vi "MB Ethernet Example Master.vi"() -> ()   [LabVIEW 2019, in "NI_modbus_upd.lvlib"]
uses:
  NI_modbus_upd.lvlib
  Ctl/MB Modbus Command.ctl
  TCP/TCP.lvclass
panel:
  out "error out":errorcluster
  in  "Remote Port":u16=502
  in  "Remote IP Address":string="127.0.0.1"
  in  "Stop":bool
  out "Slave Input Registers":u16[](array[numeric]) caption="Slave Input Registers (Read Only)"
  out "Slave Discrete Inputs":bool[](array[boolean])
  in  "Coils to Write":bool[](array[boolean])=[FALSE, FALSE, FALSE, FALSE]
  in  "Registers to Write":u16[](array[numeric])=[0, 0, 0, 0]
  # "MB Ethernet Example Master.vi\n\nInstructions\n1. Run MB Ethernet Example Slave.vi\n2. Run this VI.\n3. Modify the discrete inputs or input registers on the slave -> they're updated on the master.\n4. Modify the coils and registers on the master -> they're updated on the slave."
  # "Data to write to the slave"
  # "Slave Read-only Registers"
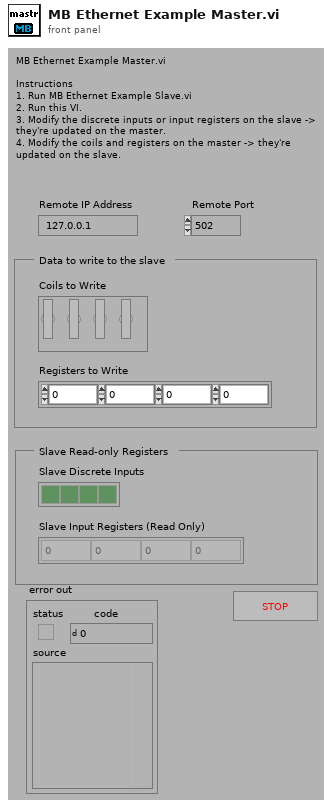
[diagram p1: front panel]
types:
  T1 = typedef "NI_modbus_upd.lvlib/MB Modbus Command.ctl" = cluster{"Function Code":u8, "Starting Address":u16, "Quantity":u16, "Data":u16[], "Discrete":bool[]}
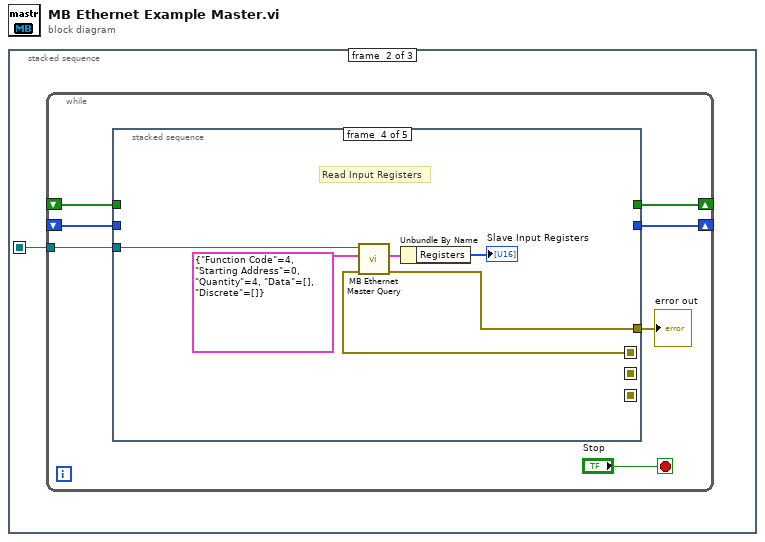
[diagram p0: block diagram]
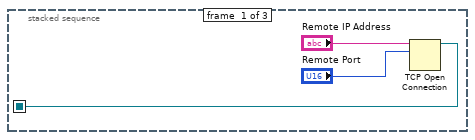
[diagram p2: hidden frame]
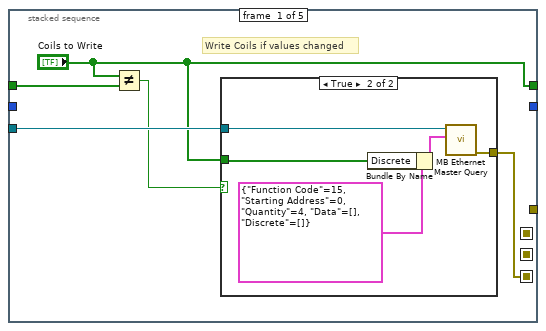
[diagram p3: hidden frame]
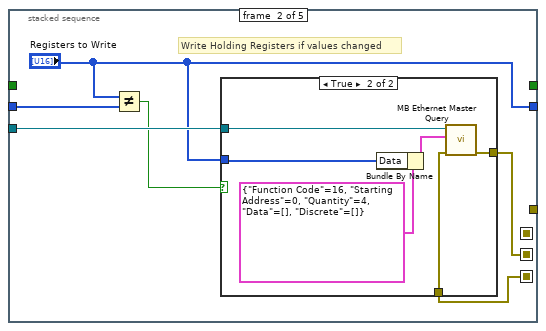
[diagram p5: hidden frame]
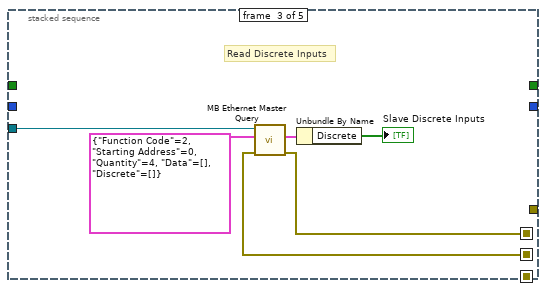
[diagram p7: hidden frame]
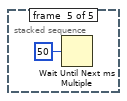
[diagram p8: hidden frame]
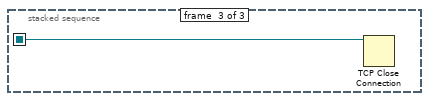
[diagram p9: hidden frame]
diagram:
  n1 = stacked-sequence {
    seq-local: [w1 _ _] -> [_ w4 w48]
    frame #0 {
      n2 = TCP Open Connection(address="Remote IP Address", remote port or service name="Remote Port") -> (connection ID=w1:refnum<k5>)  [unwired: 3 in, 1 out]
    }
    frame #1 {
      n3 = while {
        tunnel: w4 -> [w11]
        shift-right: [w9] -> _
        shift-left: _ -> [w10]
        shift-right: [w7] -> _
        shift-left: _ -> [w8]
        stop <- "Stop" stop-if-true
        n4 = stacked-sequence {
          seq-local: [w12 _ _ _ _] -> [_ w23 _ _ _]
          seq-local: [_ w22 _ _ _] -> [_ _ w36 _ _]
          seq-local: [_ _ w35 _ _] -> [_ _ _ w42 _]
          tunnel: w11 -> [w16 w27 w40 w46 _]
          tunnel: w10 -> [w15 _ _ _ _]
          tunnel: ["Coils to Write" _ _ _ _] -> w9
          tunnel: w8 -> [_ w25 _ _ _]
          tunnel: [_ "Registers to Write" _ _ _] -> w7
          tunnel: [_ _ _ w41 _] -> w5
          frame #0 {
            # "Write Coils if values changed"
            n5 = Not Equal?(x="Coils to Write", y=w15) -> (x != y?=w13:bool)
            n6 = case shown="True" w13 {
              tunnel: w16 -> [_ w19]
              tunnel: "Coils to Write" -> [_ w18]
              tunnel: [_ w17] -> w12
              frame False {
              }
              frame True {
                n7 = Bundle By Name(cluster=T1 {"Function Code"=15, "Starting Address"=0, "Quantity"=4, "Data"=[], "Discrete"=[]} ("MODBUS Command"), "Discrete"=w18) -> (w20:T1)
                n8 = call "MB Ethernet Master Query.vi"("Modbus Command"=w20, "TCP in"=w19) -> ("error out"=w17:errorcluster)  [unwired: 6 in, 3 out]
              }
            }
          }
          frame #1 {
            # "Write Holding Registers if values changed"
            n9 = Not Equal?(x="Registers to Write", y=w25) -> (x != y?=w26:bool)
            n10 = case shown="True" w26 {
              tunnel: w27 -> [_ w32]
              tunnel: "Registers to Write" -> [_ w31]
              tunnel: w23 -> [w28 w30]
              tunnel: [w28 w29] -> w22
              frame False {
              }
              frame True {
                n11 = Bundle By Name(cluster=T1 {"Function Code"=16, "Starting Address"=0, "Quantity"=4, "Data"=[], "Discrete"=[]} ("MODBUS Command"), "Data"=w31) -> (w33:T1)
                n12 = call "MB Ethernet Master Query.vi"("error in (no error)"=w30, "Modbus Command"=w33, "TCP in"=w32) -> ("error out"=w29:errorcluster)  [unwired: 5 in, 3 out]
              }
            }
          }
          frame #2 {
            # "Read Discrete Inputs"
            n13 = call "MB Ethernet Master Query.vi"("error in (no error)"=w36, "Modbus Command"=T1 {"Function Code"=2, "Starting Address"=0, "Quantity"=4, "Data"=[], "Discrete"=[]} ("MODBUS Command"), "TCP in"=w40) -> ("error out"=w35:errorcluster, "Registers"=w39:cluster{"Registers":u16[], "Discrete":bool[]})  [unwired: 5 in, 2 out]
            n14 = Unbundle By Name(w39) -> ("Discrete"=→"Slave Discrete Inputs":bool[])
          }
          frame #3 {
            # "Read Input Registers"
            n15 = call "MB Ethernet Master Query.vi"("error in (no error)"=w42, "Modbus Command"=T1 {"Function Code"=4, "Starting Address"=0, "Quantity"=4, "Data"=[], "Discrete"=[]} ("MODBUS Command"), "TCP in"=w46) -> ("error out"=w41:errorcluster, "Registers"=w45:cluster{"Registers":u16[], "Discrete":bool[]})  [unwired: 5 in, 2 out]
            n16 = Unbundle By Name(w45) -> ("Registers"=→"Slave Input Registers":u16[])
          }
          frame #4 {
            n17 = Wait Until Next ms Multiple(millisecond multiple=u32 50) -> ()  [unwired: 1 out]
          }
        }
        "error out" <- w5
      }
    }
    frame #2 {
      n18 = TCP Close Connection(connection ID=w48) -> ()  [unwired: 2 in, 2 out]
    }
  }
